vi "aryapp.vi"() -> ()   [LabVIEW 2022 SP3]
panel:
  out "Visited Positions Array":bool[][](array[boolean])=[[TRUE, TRUE, TRUE], [TRUE, FALSE, TRUE], [TRUE, TRUE, TRUE]]
  in  "右":bool
  in  "左":bool
  in  "上":bool
  in  "下":bool
  in  "Stop":bool
  in  "列":dbl
  in  "行":dbl
  out "Current Position Array":bool[][](array[boolean])=[[TRUE, TRUE, TRUE], [TRUE, FALSE, TRUE], [TRUE, TRUE, TRUE]]
  out "Boolean":bool=TRUE
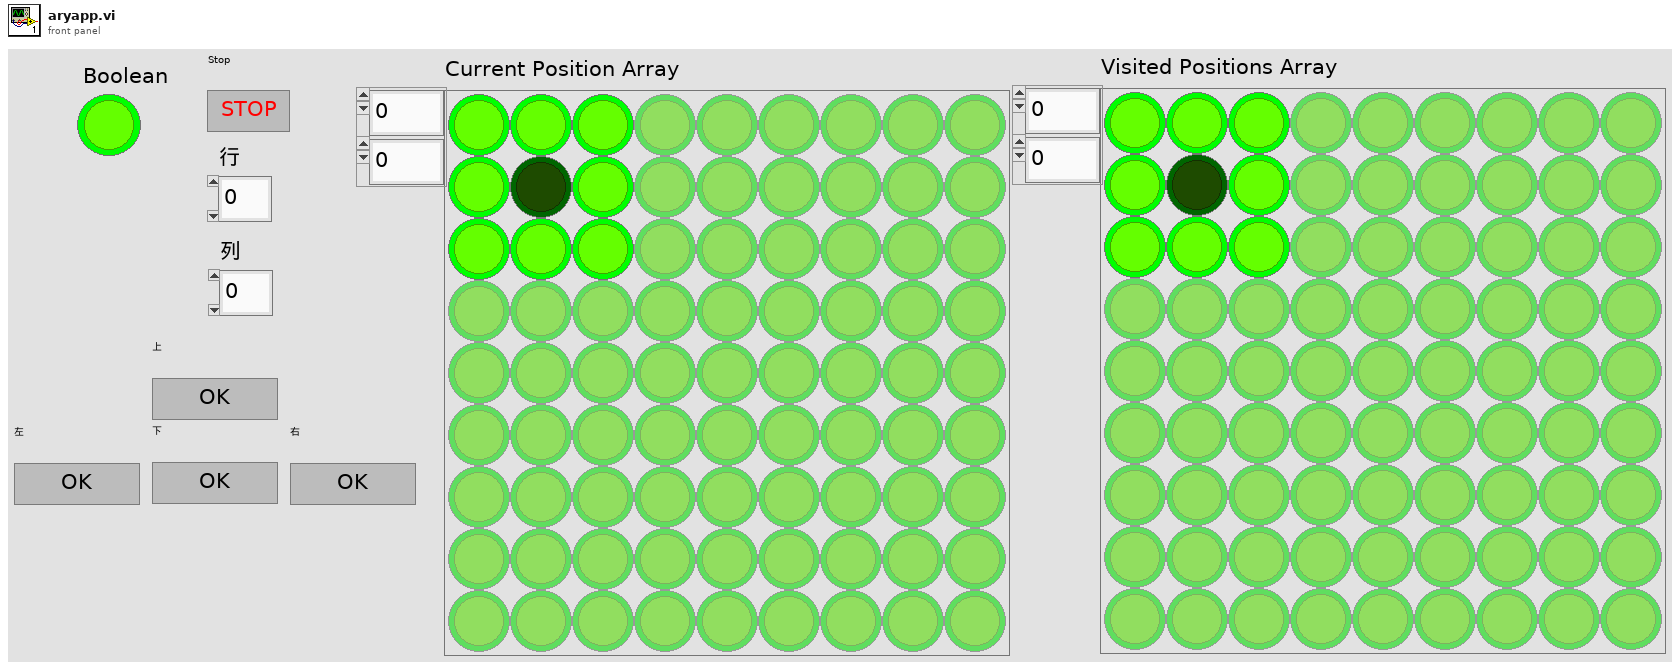
[diagram p1: front panel]
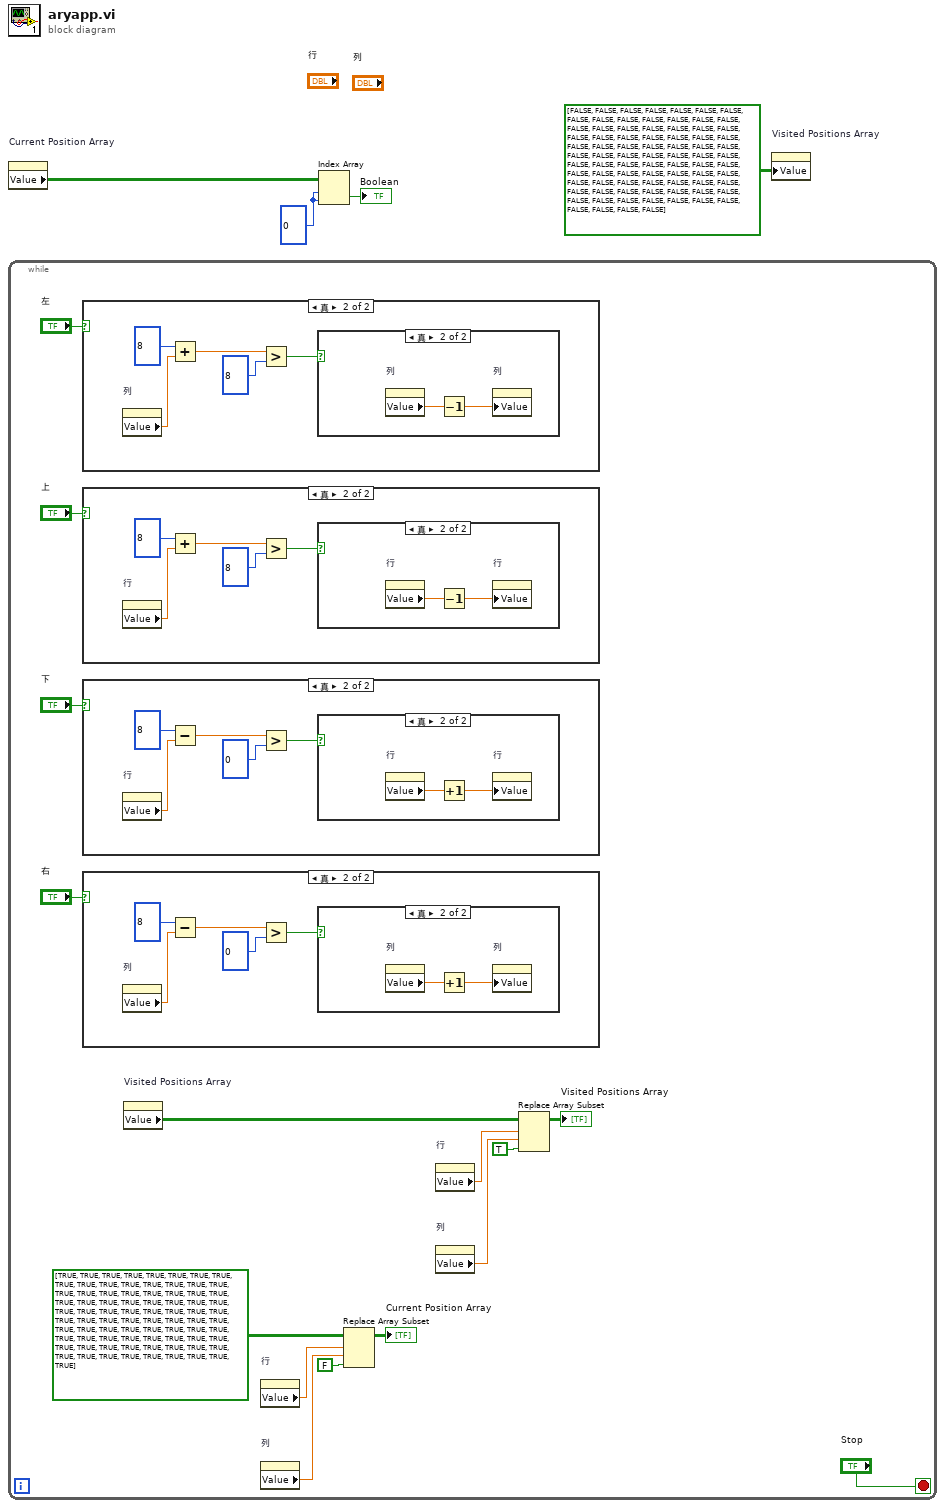
[diagram p0: block diagram]
diagram:
  w4 = 0
  n1 = property on="Current Position Array" class="Arr (严格)"() -> ("Value"=w2:bool[][])  [unwired: 2 in, 2 out]
  n2 = while {
    stop <- "Stop" stop-if-true
    n3 = case shown="真" "左" {
      frame False {
      }
      frame True {
        n4 = property on="列" class="DigNum (严格)"() -> ("Value"=w27:dbl)  [unwired: 2 in, 2 out]
        n5 = Add(x=8, y=w27) -> (x+y=w29:dbl)
        n6 = Greater?(x=w29, y=8) -> (0:w30:bool)
        n7 = case shown="真" w30 {
          frame False {
          }
          frame True {
            n8 = property on="列" class="DigNum (严格)"() -> ("Value"=w33:dbl)  [unwired: 2 in, 2 out]
            n9 = Decrement(x=w33) -> (x-1=w32:dbl)
            n10 = property on="列" class="DigNum (严格)"("Value"=w32) -> ()  [unwired: 2 in, 2 out]
          }
        }
      }
    }
    n11 = case shown="真" "上" {
      frame False {
      }
      frame True {
        n12 = property on="行" class="DigNum (严格)"() -> ("Value"=w34:dbl)  [unwired: 2 in, 2 out]
        n13 = Add(x=8, y=w34) -> (x+y=w36:dbl)
        n14 = Greater?(x=w36, y=8) -> (0:w37:bool)
        n15 = case shown="真" w37 {
          frame False {
          }
          frame True {
            n16 = property on="行" class="DigNum (严格)"() -> ("Value"=w40:dbl)  [unwired: 2 in, 2 out]
            n17 = Decrement(x=w40) -> (x-1=w39:dbl)
            n18 = property on="行" class="DigNum (严格)"("Value"=w39) -> ()  [unwired: 2 in, 2 out]
          }
        }
      }
    }
    n19 = case shown="真" "下" {
      frame False {
      }
      frame True {
        n20 = property on="行" class="DigNum (严格)"() -> ("Value"=w41:dbl)  [unwired: 2 in, 2 out]
        n21 = Subtract(x=8, y=w41) -> (x-y=w43:dbl)
        n22 = Greater?(x=w43, y=0) -> (0:w44:bool)
        n23 = case shown="真" w44 {
          frame False {
          }
          frame True {
            n24 = property on="行" class="DigNum (严格)"() -> ("Value"=w47:dbl)  [unwired: 2 in, 2 out]
            n25 = Increment(x=w47) -> (x+1=w46:dbl)
            n26 = property on="行" class="DigNum (严格)"("Value"=w46) -> ()  [unwired: 2 in, 2 out]
          }
        }
      }
    }
    n27 = case shown="真" "右" {
      frame False {
      }
      frame True {
        n28 = property on="列" class="DigNum (严格)"() -> ("Value"=w20:dbl)  [unwired: 2 in, 2 out]
        n29 = Subtract(x=8, y=w20) -> (x-y=w22:dbl)
        n30 = Greater?(x=w22, y=0) -> (0:w23:bool)
        n31 = case shown="真" w23 {
          frame False {
          }
          frame True {
            n32 = property on="列" class="DigNum (严格)"() -> ("Value"=w26:dbl)  [unwired: 2 in, 2 out]
            n33 = Increment(x=w26) -> (x+1=w25:dbl)
            n34 = property on="列" class="DigNum (严格)"("Value"=w25) -> ()  [unwired: 2 in, 2 out]
          }
        }
      }
    }
    n35 = property on="Visited Positions Array" class="Arr (严格)"() -> ("Value"=w5:bool[][])  [unwired: 2 in, 2 out]
    n36 = property on="行" class="DigNum (严格)"() -> ("Value"=w16:dbl)  [unwired: 2 in, 2 out]
    n37 = property on="列" class="DigNum (严格)"() -> ("Value"=w15:dbl)  [unwired: 2 in, 2 out]
    n38 = Replace Array Subset(array=bool[][] [[TRUE, TRUE, TRUE, TRUE, TRUE, TRUE, TRUE, TRUE, TRUE], [TRUE, TRUE, TRUE, TRUE, TRUE, TRUE, TRUE, TRUE, TRUE], [TRUE, TRUE, TRUE, TRUE, TRUE, TRUE, TRUE, TRUE, TRUE], [TRUE, TRUE, TRUE, TRUE, TRUE, TRUE, TRUE, TRUE, TRUE], [TRUE, TRUE, TRUE, TRUE, TRUE, TRUE, TRUE, TRUE, TRUE], [TRUE, TRUE, TRUE, TRUE, TRUE, TRUE, TRUE, TRUE, TRUE], [TRUE, TRUE, TRUE, TRUE, TRUE, TRUE, TRUE, TRUE, TRUE], [TRUE, TRUE, TRUE, TRUE, TRUE, TRUE, TRUE, TRUE, TRUE], [TRUE, TRUE, TRUE, TRUE, TRUE, TRUE, TRUE, TRUE, TRUE]], new element=FALSE, index (row)=w16, index (col)=w15) -> (→"Current Position Array":bool[][])
    n39 = property on="行" class="DigNum (严格)"() -> ("Value"=w7:dbl)  [unwired: 2 in, 2 out]
    n40 = property on="列" class="DigNum (严格)"() -> ("Value"=w6:dbl)  [unwired: 2 in, 2 out]
    n41 = Replace Array Subset(array=w5, new element=TRUE, index (row)=w7, index (col)=w6) -> (→"Visited Positions Array":bool[][])
  }
  n42 = Index Array(array=w2, index (row)=w4, index (col)=w4) -> (element=→"Boolean":bool)
  n43 = property on="Visited Positions Array" class="Arr (严格)"("Value"=bool[][] [[FALSE, FALSE, FALSE, FALSE, FALSE, FALSE, FALSE, FALSE, FALSE], [FALSE, FALSE, FALSE, FALSE, FALSE, FALSE, FALSE, FALSE, FALSE], [FALSE, FALSE, FALSE, FALSE, FALSE, FALSE, FALSE, FALSE, FALSE], [FALSE, FALSE, FALSE, FALSE, FALSE, FALSE, FALSE, FALSE, FALSE], [FALSE, FALSE, FALSE, FALSE, FALSE, FALSE, FALSE, FALSE, FALSE], [FALSE, FALSE, FALSE, FALSE, FALSE, FALSE, FALSE, FALSE, FALSE], [FALSE, FALSE, FALSE, FALSE, FALSE, FALSE, FALSE, FALSE, FALSE], [FALSE, FALSE, FALSE, FALSE, FALSE, FALSE, FALSE, FALSE, FALSE], [FALSE, FALSE, FALSE, FALSE, FALSE, FALSE, FALSE, FALSE, FALSE]]) -> ()  [unwired: 2 in, 2 out]
